vi "Data Producer Worker Template_Worker.vi"(0 "Data Queue":T1, 5 "Instrument Reference":refnum<k5>) -> ()   [LabVIEW 2013, in "Data Producer Worker Template.lvclass"]
uses:
  Data Producer Worker Template.lvclass
  Data Producer Worker Template_Data Queue.ctl
panel:
  out "Iteration":i32
  out "Messages Sent":i32
  # "Inputs"
  # "Debug"
  # "Outputs"
  # "This asynchronous worker has no outputs"
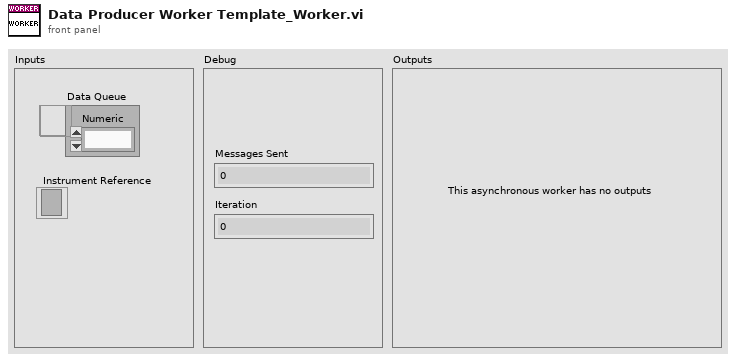
[diagram p1: front panel]
types:
  T1 = typedef "Data Producer Worker Template.lvclass/Data Producer Worker Template_Data Queue.ctl" = refnum<queue>
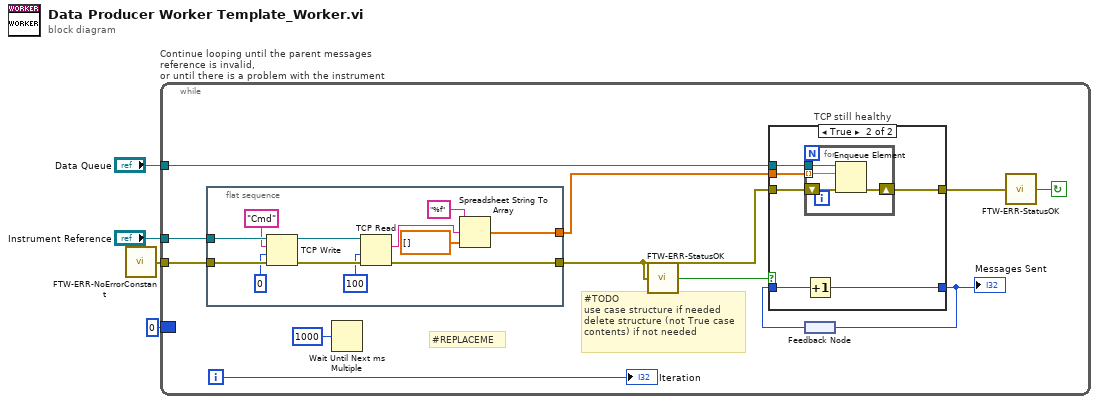
[diagram p0: block diagram]
diagram:
  n1 = call "FTW-ERR-NoErrorConstant.vi"() -> ("no error"=w3:errorcluster)
  n2 = while "Continue looping until the parent messages reference is invalid,\nor until there is a problem with the instrument" {
    border: 0 ("Messages Handled") -> [_]
    tunnel: "Data Queue" -> [w12]
    tunnel: w3 -> [w8]
    tunnel: "Instrument Reference" -> [w9]
    i -> [w15]
    stop <- w11 continue-if-true
    # "#REPLACEME"
    # "#TODO\nuse case structure if needed\ndelete structure (not True case\ncontents) if not needed"
    n3 = flat-sequence {
      tunnel: w9 -> [w28]
      tunnel: w8 -> [w27]
      tunnel: [w21] -> w7
      tunnel: [w17] -> w5
      frame #0 {
        n4 = TCP Write(connection ID=w28, data in="Cmd", error in (no error)=w27, 9:0 ("timeout ms (25000)")) -> (connection ID out=w25:refnum<k5>, error out=w26:errorcluster)  [unwired: 1 out]
        n5 = TCP Read(connection ID=w25, error in (no error)=w26, 9:100 ("timeout ms (25000)")) -> (data out=w19:string, error out=w21:errorcluster)  [unwired: 2 in, 1 out]
        n6 = Spreadsheet String To Array(format string="%f", spreadsheet string=w19, array type (2D Dbl)=dbl[] []) -> (array=w17:dbl[])  [unwired: 1 in]
      }
    }
    n7 = Wait Until Next ms Multiple(millisecond multiple=u32 1000) -> ()  [unwired: 1 out]
    n8 = call "FTW-ERR-StatusOK.vi"("error to check"=w7) -> ("Status OK?"=w6:bool)
    n9 = feedback #1() -> (w14:i32)
    n10 = case "TCP still healthy" shown="True" w6 {
      tunnel: w12 -> [_ w36]
      tunnel: [w30 w35] -> w13
      tunnel: w7 -> [w30 w32]
      tunnel: [w29 w34] -> w16
      tunnel: w14 -> [w29 w33]
      tunnel: w5 -> [_ w31]
      frame False {
      }
      frame True {
        n11 = for {
          tunnel: w36 -> [w40]
          shift-right: [w39] -> w35
          shift-left: w32 -> [w38]
          tunnel: w31 -> [w37] mode=indexing
          n12 = Enqueue Element(queue=w40, element=w37, error in (no error)=w38) -> (error out=w39:errorcluster)  [unwired: 1 in, 2 out]
        }
        n13 = Increment(x=w33) -> (x+1=w34:i32)
      }
    }
    "Messages Sent" <- w16
    n14 = feedback-in #1(w16) -> ()
    n15 = call "FTW-ERR-StatusOK.vi"("error to check"=w13) -> ("Status OK?"=w11:bool)
    "Iteration" <- w15
  }
